vi "Create.vi"(7 "mode settings":variant, 8 "error in":errorcluster, 9 "number of default channels":i32, 10 "channel settings":variant, 11 "digital input mode in":refnum<class "Digital Input and Output Mode.lvclass">) -> (0 "error out":errorcluster, 1 "channels":refnum<class "Channel.lvclass">[](array[class]), 3 "digital input mode out":refnum<class "Digital Input and Output Mode.lvclass">)   [LabVIEW 2017, in "Scan Engine Scripting.lvlib" / "Digital Input and Output Mode.lvclass"]
uses:
  Digital Input and Output Mode.lvclass
  Channel Classes/Channel/Channel.lvclass
  Digital Output Mode/Digital Output Mode.lvclass
  Digital Input Mode/Digital Input Mode.lvclass
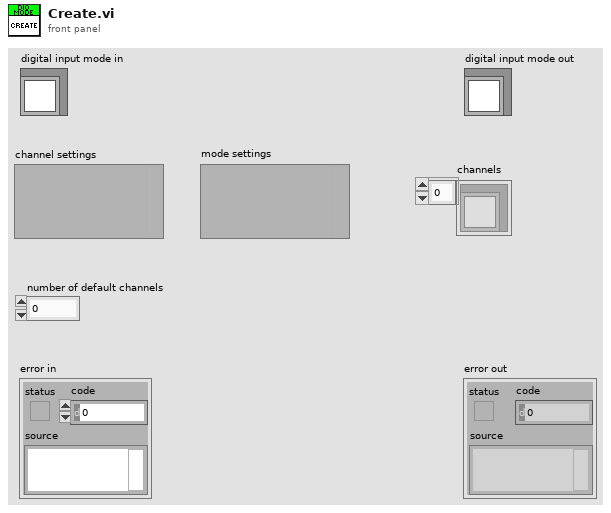
[diagram p1: front panel]
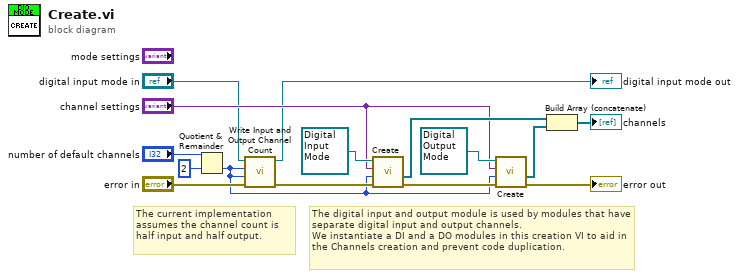
[diagram p0: block diagram]
diagram:
  # "The current implementation assumes the channel count is half input and half output."
  # "The digital input and output module is used by modules that have separate digital input and output channels.\nWe instantiate a DI and a DO modules in this creation VI to aid in the Channels creation and prevent code duplication."
  n1 = Quotient & Remainder(x="number of default channels", y=2) -> (floor(x/y)=w1:i32)  [unwired: 1 out]
  n2 = call "Write Input and Output Channel Count.vi"("error in"="error in", "Output Channels"=w1, "Input Channels"=w1, "Digital Input and Output Mode in"="digital input mode in") -> ("error out"=w2:errorcluster, "Digital Input and Output Mode out"=→"digital input mode out":refnum<class "Digital Input and Output Mode.lvclass">)  [unwired: 6 in]
  n3 = call-dynamic "Create.vi"("error in"=w2, "number of default channels"=w1, "channel settings"="channel settings", "digital input mode in"=refnum<class "Digital Input Mode.lvclass"> refnum ("Scan Engine Scripting.lvlib:Digital Input Mode.lvclass")) -> ("error out"=w8:errorcluster, "channels"=w12:refnum<class "Channel.lvclass">[])  [unwired: 5 in, 1 out]
  n4 = call-dynamic "Create.vi"("error in"=w8, "number of default channels"=w1, "channel settings"="channel settings", "digital output mode in"=refnum<class "Digital Output Mode.lvclass"> refnum ("Scan Engine Scripting.lvlib:Digital Output Mode.lvclass")) -> ("error out"=→"error out":errorcluster, "channels"=w11:refnum<class "Channel.lvclass">[])  [unwired: 5 in, 1 out]
  n5 = Build Array (concatenate)(w12, w11) -> (→"channels":refnum<class "Channel.lvclass">[])
